vi "lvEtherbone.application_example_read_write.vi"() -> ()   [LabVIEW 2009, in "lvEtherbone.lvlib"]
doc: "This example performs a multiple read/write on a Etherbone device."
uses:
  lvEtherbone.lvlib
  lvEtherbone.eb_mode_t.ctl
  lvEtherbone.lveb_status_t.ctl
panel:
  out "timed out?":bool
  out "eb_status":T1
  in  "dataW":u64[](array[numeric])=[291, 837] format="%.0x"
  in  "modeW":T2=1 items=["EB_UNDEFINED"=-1, "EB_FIFO"=0, "EB_LINEAR"=1]
  in  "addressW":u64=32783 format="%.0x"
  in  "nR":i32=2
  in  "modeR":T2=1 items=["EB_UNDEFINED"=-1, "EB_FIFO"=0, "EB_LINEAR"=1]
  out "dataR":u64[](array[numeric]) format="%.0x"
  in  "addressR":u64=32768 format="%.0x"
  in  "timeout [ms]":i32=1000
  in  "ip_port":string="111.222.333.444:5555"
  out "error out":errorcluster
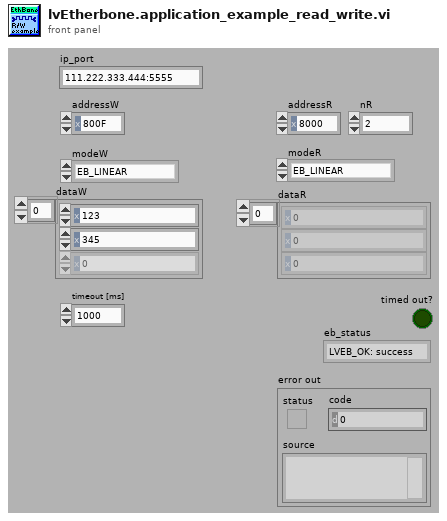
[diagram p1: front panel]
types:
  T1 = typedef "lvEtherbone.lvlib/lvEtherbone.lveb_status_t.ctl" = enum32{"LVEB_OK: success", "LVEB_UNKNOWN: unknown error", "LVEB_OS: operating system forbids access", "LVEB_PORT: port in use or unavailable", "LVEB_ID: ID invalid or out of resources", "LVEB_SOCKET: socket invalid or unavailable", "LVEB_EB: remote address is not Etherbone conformant", "LVEB_IP: bad format or network address", "LVEB_PORTWIDTH: port width error", "LVEB_DEVICEBUSY: Etherbone device still busy", "LVEB_DEVICEFAIL: operation on Wishbone device failed", "LVEB_DEVICEEXIST: Etherbone device already exists, overlaps, or does not exist", "LVEB_TIMEDOUT: a timeout occurred", "LVEB_OVERFLOW: payload of Etherbone exceeded", "LVEB_ADDRESS: bad address", "LVEB_ADDRESSWIDTH: address width error"}
  T2 = typedef "lvEtherbone.lvlib/lvEtherbone.eb_mode_t.ctl" = i32
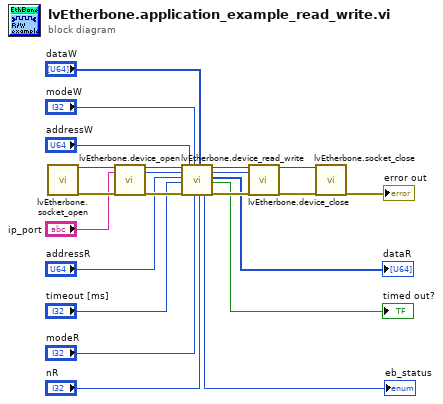
[diagram p0: block diagram]
diagram:
  n1 = call "lvEtherbone.socket_open.vi"() -> ("eb_socket_ID"=w20:i32, "error out"=w21:errorcluster)  [unwired: 17 in, 1 out]
  n2 = call "lvEtherbone.device_open.vi"("eb_socket_ID"=w20, "ip_port"="ip_port", "error in (no error)"=w21) -> ("eb_socket_ID out"=w13:i32, "eb_device_ID"=w17:i32, "error out"=w19:errorcluster)  [unwired: 12 in, 2 out]
  n3 = call "lvEtherbone.device_read_write.vi"("eb_socket_ID"=w13, "eb_device_ID"=w17, "addressR"="addressR", "timeout [ms]"="timeout [ms]", "error in (no error)"=w19, "addressW"="addressW", "modeW"="modeW", "modeR"="modeR", "dataW"="dataW", "nR"="nR") -> ("eb_status"=→"eb_status":T1, "eb_socket_ID out"=w12:i32, "eb_device_ID out"=w10:i32, "dataR"=→"dataR":u64[], "timed out?"=→"timed out?":bool, "error out"=w18:errorcluster)  [unwired: 4 in]
  n4 = call "lvEtherbone.device_close.vi"("eb_socket_ID"=w12, "eb_device_ID"=w10, "error in (no error)"=w18) -> ("eb_socket_ID out"=w11:i32, "error out"=w16:errorcluster)  [unwired: 14 in, 1 out]
  n5 = call "lvEtherbone.socket_close.vi"("eb_socket_ID"=w11, "error in (no error)"=w16) -> ("error out"=→"error out":errorcluster)  [unwired: 16 in, 1 out]
